vi "parser.vi"(8 "error in":errorcluster, 11 "входная посылка":string) -> (0 "error out":errorcluster, 1 "температура":string, 2 "Парсер: скорость":i32, 3 "Парсер: канал":i32)   [LabVIEW 2014]
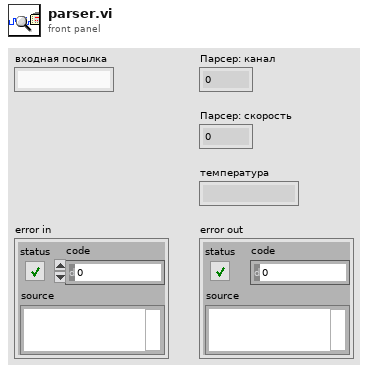
[diagram p1: front panel]
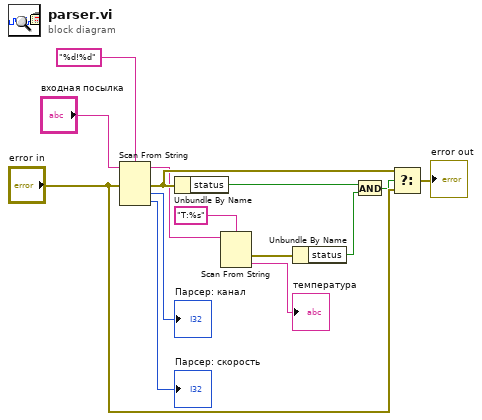
[diagram p0: block diagram]
diagram:
  n1 = Scan From String(format string="%d!%d" ("regular expression"), input string="входная посылка", error in="error in") -> (remaining string=w10:string, error out=w11:errorcluster, output 1=→"Парсер: канал":i32, output 2=→"Парсер: скорость":i32)  [unwired: 3 in, 1 out]
  n2 = Unbundle By Name(w11) -> ("status"=w6:bool)
  n3 = Scan From String(format string="T:%s" ("regular expression"), input string=w10) -> (error out=w9:errorcluster, output 1=→"температура":string)  [unwired: 3 in, 2 out]
  n4 = Unbundle By Name(w9) -> ("status"=w7:bool)
  n5 = And(x=w6, y=w7) -> (x .and. y?=w8:bool)
  n6 = Select(t=w11, s=w8, f="error in") -> (s? t:f=→"error out":errorcluster)
